vi "ListBox_Display Selected Tests in Order.vi"(8 "Error In":errorcluster, 10 "Tests":string, 11 "Meas_Type_exp1":refnum<vi>) -> (0 "Error Out":errorcluster, 2 "Item Names":string[](array[string]), 3 "Values":i32[](array[numeric]))   [LabVIEW 2013]
uses:
  Controls/Test Selection.ctl
  <vilib>/Utility/config.llb/Read Key (String).vi
  <userlib>/_OpenG.lib/array/array.llb/Remove Duplicates from 1D Array (String)__ogtk.vi
  <vilib>/Utility/config.llb/NI_LVConfig.lvlib
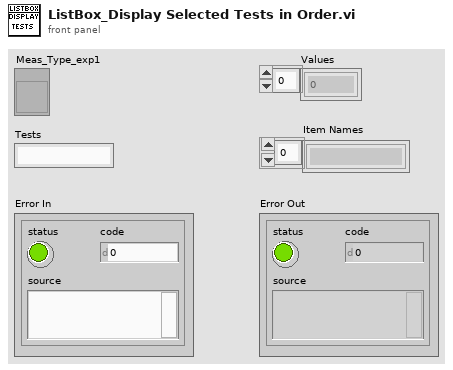
[diagram p1: front panel]
types:
  T1 = typedef "NI_LVConfig.lvlib/Config Data RefNum.ctl" = refnum<k1>
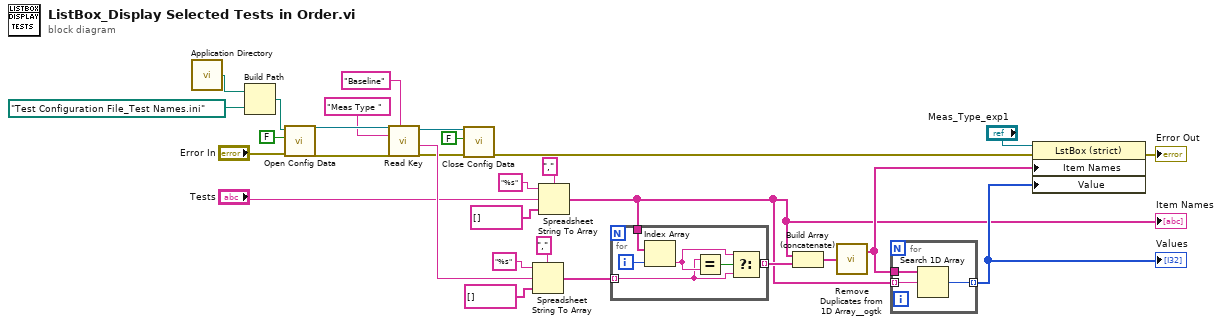
[diagram p0: block diagram]
diagram:
  n1 = call <vilib>:"Application Directory.vi"() -> ("Application Directory"=w23:path)
  n2 = Build Path(base path=w23, name or relative path=path "Test Configuration File_Test Names.ini" ("default name")) -> (appended path=w24:path)
  n3 = call <vilib>:"Open Config Data.vi"("error in (no error)"="Error In", "create file if necessary (T)"=FALSE ("create file if necessary? (T)"), "configuration file path"=w24) -> ("error out"=w21:errorcluster, "refnum"=w22:T1)  [unwired: 6 in, 1 out]
  n4 = call-poly <vilib>:"Read Key.vi"("section"="Baseline", "error in (no error)"=w21, "key"="Meas Type " ("Key 1"), "refnum"=w22) -> ("error out"=w15:errorcluster, "value"=w18:string, "refnum out"=w14:T1)  [unwired: 4 in, 1 out]
  n5 = call <vilib>:"Close Config Data.vi"("error in (no error)"=w15, "write file if changed (T)"=FALSE ("write configuration file? (T)"), "refnum"=w14) -> ("error out"=w6:errorcluster)  [unwired: 8 out]
  n6 = Spreadsheet String To Array(delimiter (Tab)=",", format string="%s", spreadsheet string=w18, array type (2D Dbl)=string[] []) -> (array=w17:string[])
  n7 = Spreadsheet String To Array(delimiter (Tab)=",", format string="%s", spreadsheet string="Tests", array type (2D Dbl)=string[] []) -> (array=w1:string[])
  "Item Names" <- w1
  n8 = for {
    tunnel: w17 -> [w30] mode=indexing
    tunnel: w1 -> [w35]
    tunnel: [w32] -> w12 mode=indexing
    i -> [w34]
    n9 = Index Array(array=w35, index=w34) -> (element=w31:string)
    n10 = Equal?(x=w30, y=w31) -> (x = y?=w33:bool)
    n11 = Select(t=w31, s=w33, f=w30) -> (s? t:f=w32:string)
  }
  n12 = Build Array (concatenate)(w1, w12) -> (w13:string[])
  n13 = call-poly <userlib>:"Remove Duplicates from 1D Array__ogtk.vi"("Input Array"=w13) -> ("Output Array"=w8:string[])  [unwired: 1 out]
  n14 = for {
    tunnel: w8 -> [w38]
    tunnel: w1 -> [w37] mode=indexing
    tunnel: [w36] -> w7 mode=indexing
    n15 = Search 1D Array(1D array=w38, element=w37) -> (index of element=w36:i32)  [unwired: 1 in]
  }
  "Values" <- w7
  n16 = property class="LstBox (strict)"(reference="Meas_Type_exp1", error in=w6, "Item Names"=w8, "Value"=w7) -> (error out=→"Error Out":errorcluster)  [unwired: 1 out]
